vi "mxwScript_API_Option_SetStartDiagram(Reference).vi"(7 "Frame":u32, 8 "error in (no error)":errorcluster, 10 "structureRef in":refnum<vi>, 11 "options in":T1[](array[typedef])) -> (0 "error out":errorcluster, 2 "structureRef out":refnum<vi>, 3 "options out":T1[](array[typedef]))   [LabVIEW 2017]
doc: "Sets the password so password protected VIs can be generated into."
uses:
  codeGenAPISupport.llb/cgAPI_mxwScript_OptionData.ctl
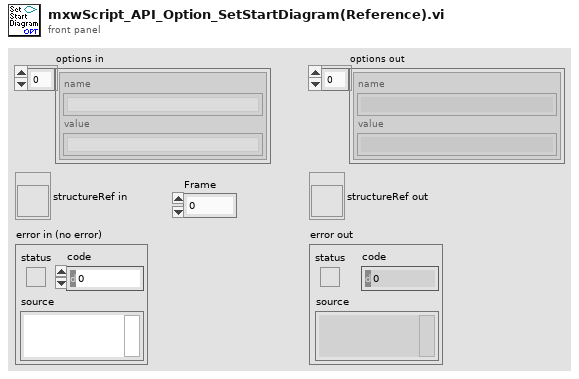
[diagram p1: front panel]
types:
  T1 = typedef "cgAPI_mxwScript_OptionData.ctl" = cluster{"name":string, "value":string}
  T2 = typedef "LVPositionTypeDef.ctl" = cluster{"Left":i32, "Top":i32}
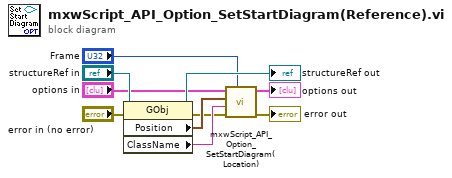
[diagram p0: block diagram]
diagram:
  n1 = property class="GObj"(reference="structureRef in", error in="error in (no error)") -> (reference out=→"structureRef out":refnum<vi>, error out=w2:errorcluster, "Position"=w3:T2, "ClassName"=w5:string)
  n2 = call "mxwScript_API_Option_SetStartDiagram(Location).vi"("options in"="options in", "Position"=w3, "ClassName"=w5, "error in (no error)"=w2, "Frame"="Frame") -> ("options out"=→"options out":T1[], "error out"=→"error out":errorcluster)  [unwired: 4 in]
